vi "DHE_Get.vi"(0 "refnum":i32, 1 "DHE_DBSRef":T1, 2 "Command + switches":string, 5 "Command":string, 7 "physical unit":string, 9 "swhitches":string[](array[string]), 11 "error in (no error)":errorcluster) -> (4 "refnum out":i32, 6 "response":string, 15 "error out":errorcluster)   [LabVIEW 2016]
uses:
  Common/public/vis/CMN_TimingInfo.ctl
  DBSHAND/private/vis/DatabaseHand_RefNum.ctl
  DBSHAND/private/vis/DatabaseHand_Element_Get(string).vi
  DBSHAND/private/vis/DatabaseHand_Element_Get(U32).vi
  DBSHAND/private/vis/DatabaseHand_Element_Get(bool).vi
  DBSHAND/private/vis/DatabaseHand_Element_Get(double).vi
  DBSHAND/private/vis/DatabaseHand_Element_Set(I32).vi
  DBSHAND/private/vis/DatabaseHand_Element_Get(I32).vi
panel:
  out "Timing":T2={"PixelTime"=1.0, "SkipPixel"=1.0, "SkipRow"=1.0, "ShiftRow"=1.0, "ShiftedPix"=1, "known_overhead"=1.0, "DET_READ_TIME"=1.0} {"DET_READ_TIME" format="%.2f"; "known_overhead" format="%.2f"; "ShiftRow" format="%.2f"; "SkipRow" format="%.2f"; "SkipPixel" format="%.2f"; "PixelTime" format="%.2f"}
  out "ControllerConfigCluster":T3
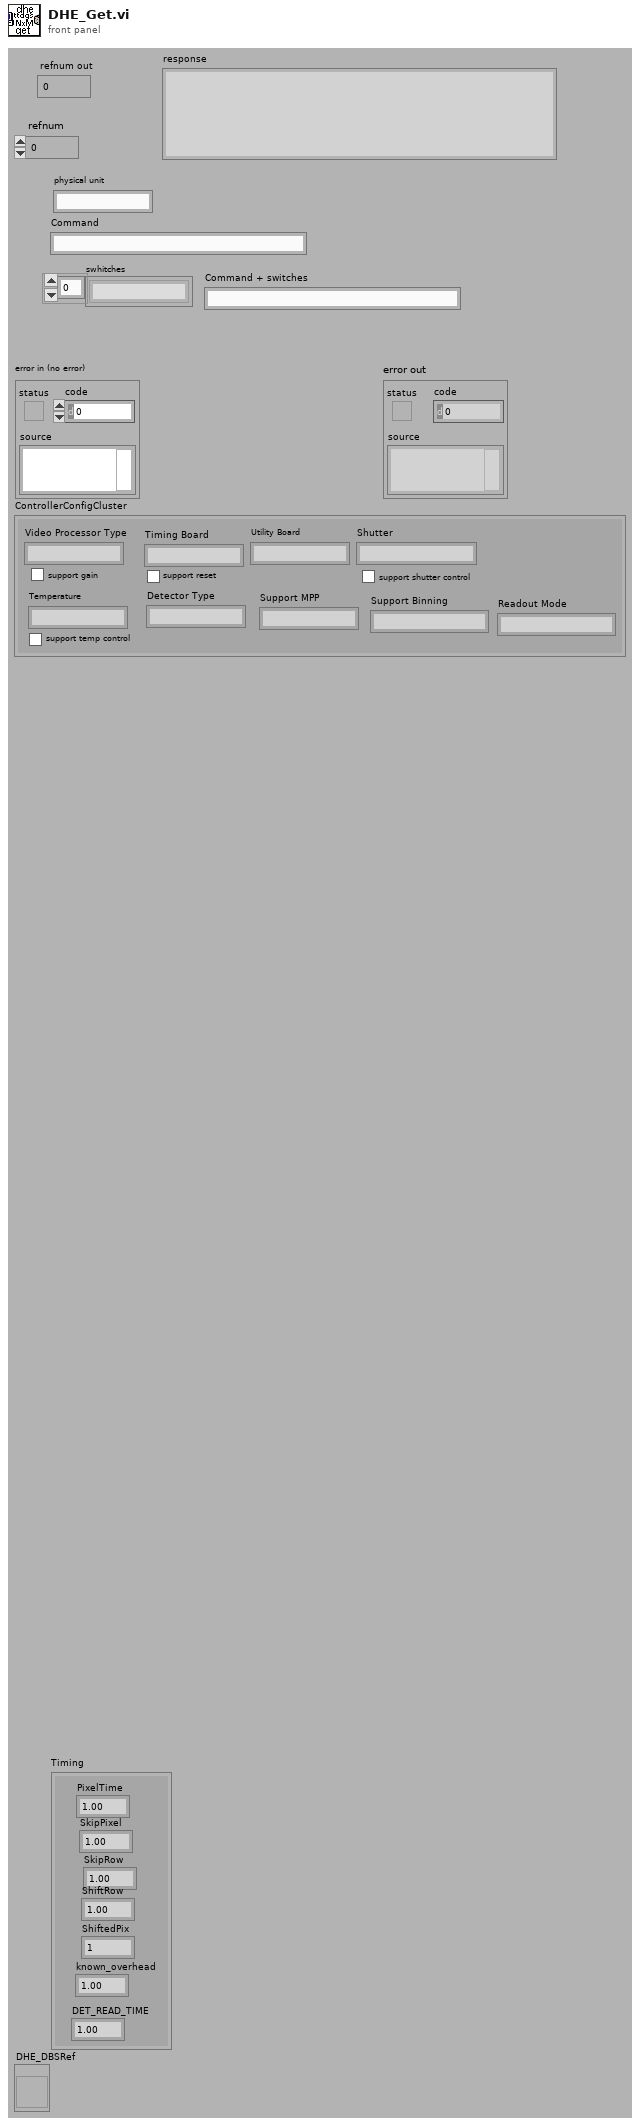
[diagram p1: front panel]
types:
  T1 = typedef "DatabaseHand_RefNum.ctl" = refnum<vi>
  T2 = typedef "CMN_TimingInfo.ctl" = cluster{"PixelTime":sgl, "SkipPixel":sgl, "SkipRow":sgl, "ShiftRow":sgl, "ShiftedPix":u16, "known_overhead":sgl, "DET_READ_TIME":sgl}
  T3 = cluster{"Video Processor Type":string, "support gain":bool, "Timing Board":string, "support reset":bool, "Utility Board":string, "Shutter":string, "Temperature":string, "support temp control":bool, "Detector Type":string, "Support MPP":string, "Support Binning":string, "Readout Mode":string, "support shutter control":bool}
  T4 = enum16{"add", "delete", "find", "clear all", "getall"}
  T5 = typedef "CMN_ContStatus.ctl" = cluster{"Response":string, "power":bool, "shutter":bool, "artifdata":bool, "idlemode":bool, "reset":bool, "gain":u8, "speed":u8, "resetPCI":bool, "autoshutter":bool, "TempSetPoint":i32, "multipleextensions":bool, "displayImage":bool, "coadding":bool, "images being coadded":i32, "Operation Mode":enum16{"normal", "coadd", "fawler"}, "frames to write":cluster{"subs":bool, "reset":bool, "exposed":bool}, "fawler samples":i32, "write auto":bool, "datatype":string, "frames to display":cluster{"subs":bool, "reset":bool, "exposed":bool}, "sur":i32, "autoclear":bool}
  T6 = typedef "DHE_Obs.ctl" = cluster{"observer":string, "obstype":string, "exptime":dbl, "coadds":i32, "fowler":i32, "nimages":i32, "display":bool, "autowrite":bool, "frames to write":cluster{"subs":bool, "reset":bool, "exposed":bool}, "frames to display":cluster{"subs":bool, "reset":bool, "exposed":bool}, "sur":i32}
  T7 = typedef "DHE_Img.ctl" = cluster{"title":string, "comment":string, "rootname":string, "imnumber":i32, "mext":bool, "imdir":string, "basename":string, "imprefix":string, "imsufix":string, "froot":string}
  T8 = typedef "GEOM_AmpModifiers.ctl" = cluster{"Binning":T9, "sections":T10[]}
  T9 = typedef "GEOM_Binning.ctl" = cluster{"x":u32, "y":u32}
  T10 = typedef "GEOM_Moifier.ctl" = cluster{"name":string, "header section":string, "comment":string, "value":i32, "binning?":bool, "Where":enum16{"predata", "postdata"}, "add In":enum16{"columns", "rows", "none"}}
  T11 = enum16{"Idle", "Exposing", "Paused", "AbortExp", "Reading", "AbortRead", "FinishedReading", "Resetting", "Reducing", "Initializing"}
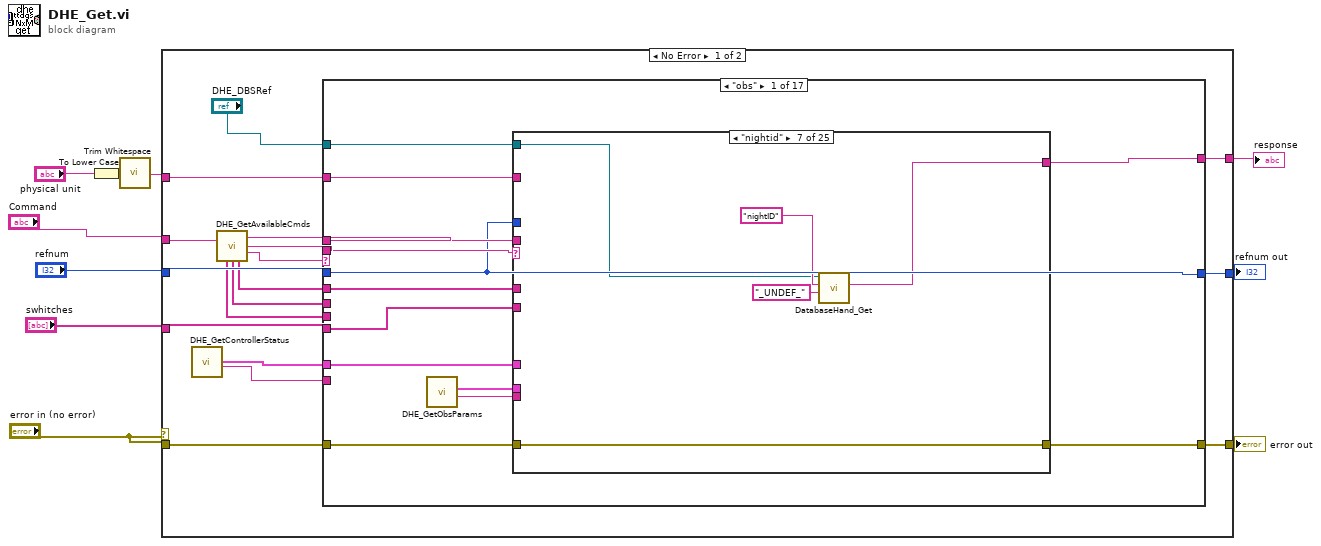
[diagram p0: block diagram]
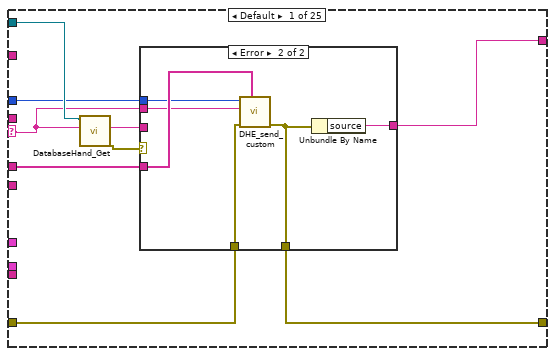
[diagram p2: hidden frame]
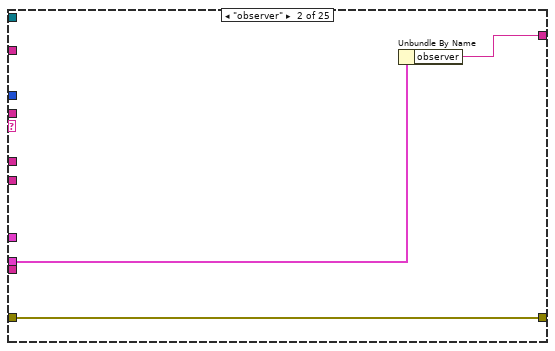
[diagram p4: hidden frame]
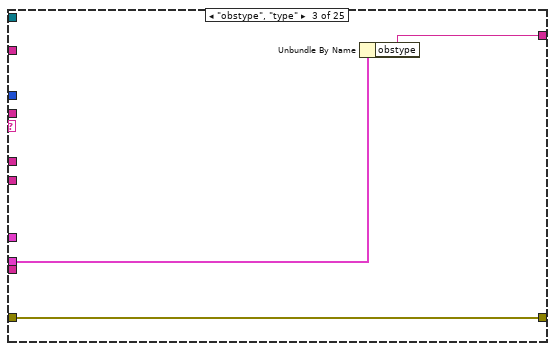
[diagram p5: hidden frame]
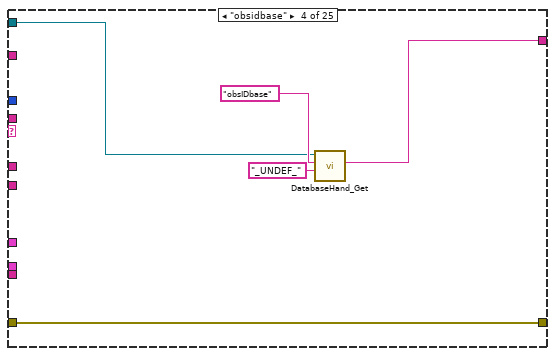
[diagram p6: hidden frame]
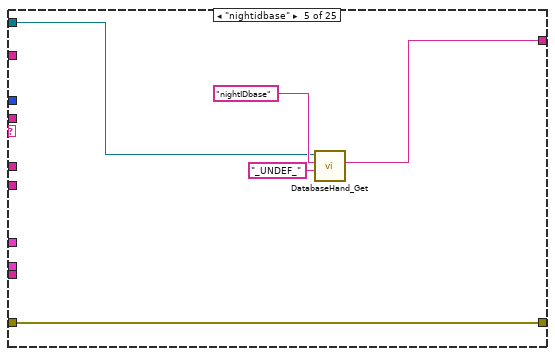
[diagram p7: hidden frame]
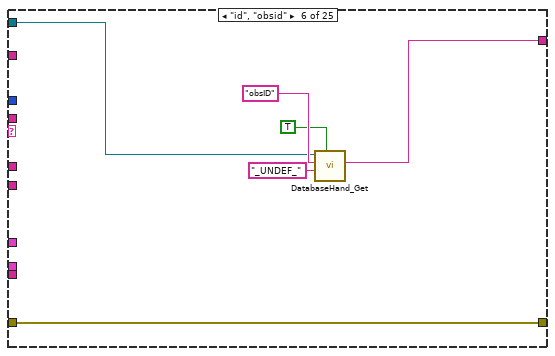
[diagram p8: hidden frame]
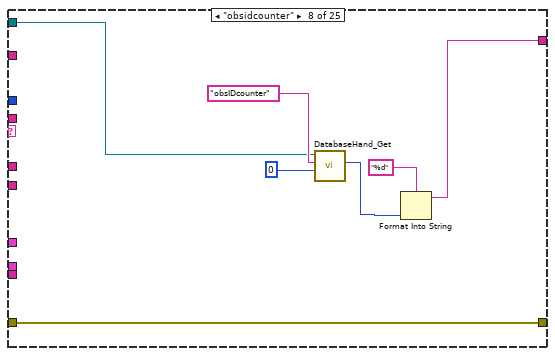
[diagram p9: hidden frame]
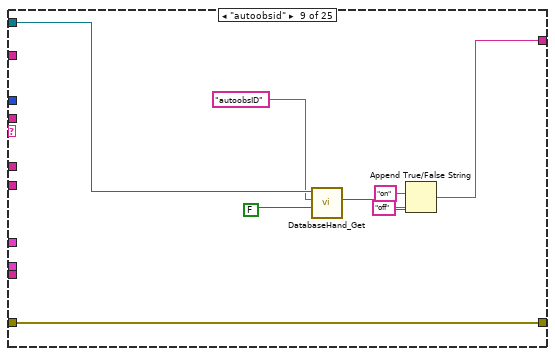
[diagram p10: hidden frame]
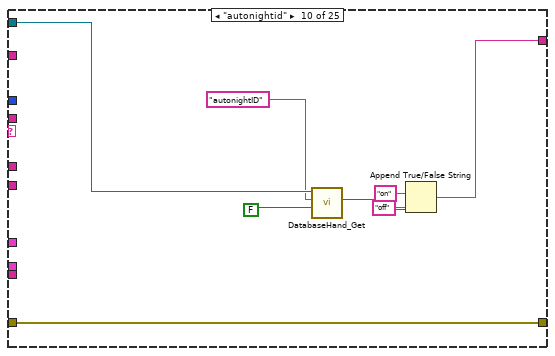
[diagram p11: hidden frame]
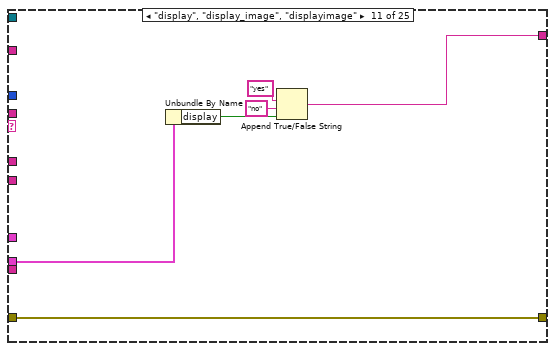
[diagram p12: hidden frame]
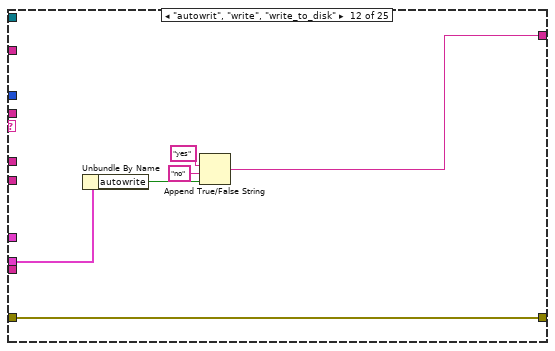
[diagram p13: hidden frame]
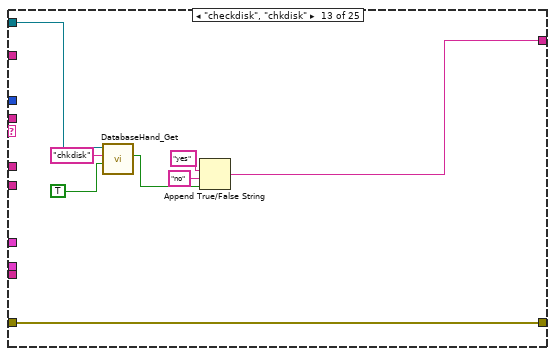
[diagram p14: hidden frame]
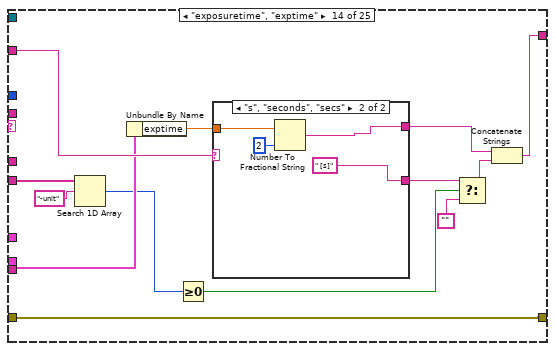
[diagram p15: hidden frame]
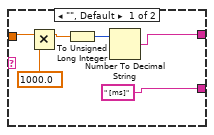
[diagram p16: hidden frame]
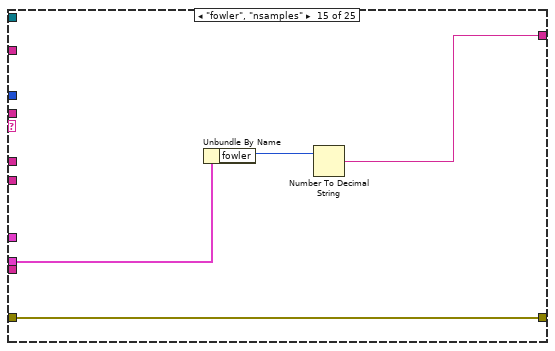
[diagram p17: hidden frame]
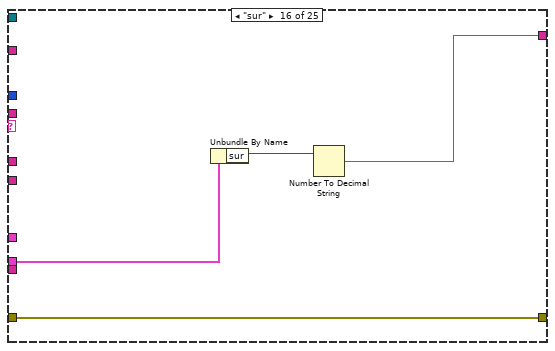
[diagram p18: hidden frame]
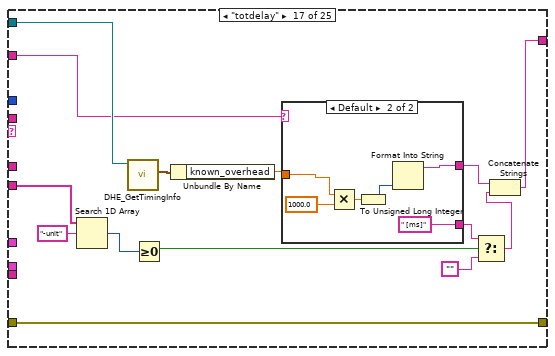
[diagram p19: hidden frame]
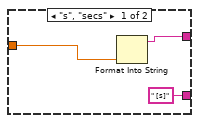
[diagram p20: hidden frame]
diagram:
  n1 = To Lower Case(string="physical unit") -> (all lower case string=w5:string)
  n2 = call <vilib>:"Trim Whitespace.vi"("string"=w5) -> ("trimmed string"=w1:string)  [unwired: 1 in]
  n3 = case shown="No Error" "error in (no error)" {
    tunnel: "error in (no error)" -> [w27 w945]
    tunnel: [w26 w945] -> w8
    tunnel: "refnum" -> [w25 w946]
    tunnel: [w24 w946] -> w10
    tunnel: "Command" -> [w19 _]
    tunnel: w1 -> [w22 _]
    tunnel: [w21 w944] -> w4
    tunnel: "swhitches" -> [w20 _]
    frame No Error {
      n4 = call "DHE_GetControllerStatus.vi"() -> ("dhe string"=w12:string, "ControllerStatus"=w23:T5)  [unwired: 10 out]
      n5 = call "DHE_GetAvailableCmds.vi"("input command"=w19) -> ("remaining"=w18:string, "field"=w16:string, "parent"=w17:string, "SDSU_image_cmds out"=w15:string[], "SDSU_dhe_cmds out"=w14:string[], "SDSU_obs_cmds out"=w13:string[])  [unwired: 9 out]
      n6 = case shown="\"obs\"" w17 {
        selector: w17 -> [_ _ _ _ _ _ _ _ _ _ _ _ _ _ _ _ w911]
        tunnel: w27 -> [w36 w261 w418 w759 w797 w802 w808 w812 w823 w841 w845 w851 w855 w864 w871 w875 w924]
        tunnel: [w35 w260 w417 w759 w797 w802 w808 w812 w822 w838 w844 w851 w855 w864 w871 w874 w923] -> w26
        tunnel: w25 -> [w29 w253 w408 w758 w796 w805 w809 w813 w821 w840 w846 w853 w854 w863 w870 w881 w921]
        tunnel: [w29 w253 w408 w758 w796 w805 w809 w813 w821 w840 w846 w853 w854 w863 w870 w881 w920] -> w24
        tunnel: w18 -> [w33 w262 w411 _ _ _ _ _ _ w837 _ w848 _ _ _ w884 w918]
        tunnel: w23 -> [w38 w259 w413 _ _ _ _ _ _ _ _ _ _ _ _ _ _]
        tunnel: w22 -> [w34 w258 _ _ _ _ _ _ _ _ _ _ _ _ _ _ _]
        tunnel: [w39 w265 w416 w757 w798 w801 w807 w811 w814 w839 w842 w852 w856 w859 w868 w876 w922] -> w21
        tunnel: w20 -> [w28 w254 w412 _ _ _ _ _ w820 _ _ _ _ _ _ w880 _]
        tunnel: w16 -> [w40 w264 w415 _ _ _ _ _ _ _ _ _ _ _ _ _ _]
        tunnel: w15 -> [_ w263 _ _ _ _ _ _ _ _ _ _ _ _ _ _ _]
        tunnel: w14 -> [_ _ w414 _ _ _ _ _ _ _ _ _ _ _ _ _ _]
        tunnel: w13 -> [w37 _ _ _ _ _ _ _ _ _ _ _ _ _ _ _ _]
        tunnel: w12 -> [_ _ w410 _ _ _ _ _ _ _ _ _ _ _ _ _ _]
        tunnel: "DHE_DBSRef" -> [w30 w255 w409 _ _ _ _ _ _ _ _ _ _ w867 w873 _ w919]
        frame "obs" {
          n7 = call "DHE_GetObsParams.vi"() -> ("obs string"=w31:string, "DHE_OBS"=w32:T6)  [unwired: 10 out]
          n8 = case shown="\"nightid\"" w40 {
            selector: w40 -> [w42 _ _ _ _ _ _ _ _ _ _ _ _ _ _ _ _ _ _ _ _ _ _ _ _]
            tunnel: [w48 w58 w61 w64 w69 w75 w80 w85 w94 w102 w110 w116 w125 w130 w153 w157 w163 w186 w208 w228 w233 w236 w237 w244 w251] -> w39
            tunnel: w38 -> [_ _ _ _ _ _ _ _ _ _ _ _ _ _ _ _ _ _ _ _ _ _ w242 w249 _]
            tunnel: w37 -> [w49 _ _ _ _ _ _ _ _ _ _ _ _ _ _ _ _ _ _ _ _ _ _ _ _]
            tunnel: w36 -> [w47 w60 w63 w65 w70 w76 w81 w89 w93 w101 w109 w115 w124 w139 w152 w156 w171 w194 w216 w227 w232 w235 w243 w250 w252]
            tunnel: [w46 w60 w63 w65 w70 w76 w81 w89 w93 w101 w109 w115 w124 w139 w152 w156 w171 w194 w216 w227 w232 w234 w243 w250 w252] -> w35
            tunnel: w34 -> [_ _ _ _ _ _ _ _ _ _ _ _ _ w140 _ _ w168 w191 w213 _ _ _ _ _ _]
            tunnel: w33 -> [_ _ _ _ _ _ _ _ _ _ _ _ _ _ _ _ _ _ _ _ _ _ _ _ _]
            tunnel: w32 -> [_ w59 w62 _ _ _ _ _ _ _ w108 w114 _ w138 w151 w155 _ _ _ w226 w231 _ _ _ _]
            tunnel: w31 -> [_ _ _ _ _ _ _ _ _ _ _ _ _ _ _ _ _ _ _ _ _ _ _ _ w251]
            tunnel: w30 -> [w44 _ _ w66 w71 w77 w82 w90 w95 w103 _ _ w123 _ _ _ w172 _ _ _ _ _ _ _ _]
            tunnel: w29 -> [w41 _ _ _ _ _ _ _ _ _ _ _ _ _ _ _ _ w193 w215 _ _ _ _ _ _]
            tunnel: w28 -> [_ _ _ _ _ _ _ _ _ _ _ _ _ w136 _ _ w166 w188 w210 _ _ _ _ _ _]
            frame Default {
              n9 = call-poly "DatabaseHand_Get.vi"("name"=w42, "Database RefNum in"=w44) -> ("error out"=w45:errorcluster, "value"=w43:string)  [unwired: 3 in, 5 out]
              n10 = case shown="Error" w45 {
                tunnel: w49 -> [_ w57]
                tunnel: [w50 w56] -> w48
                tunnel: w47 -> [w51 w55]
                tunnel: [w51 w54] -> w46
                tunnel: w42 -> [_ w53]
                tunnel: w43 -> [w50 _]
                tunnel: w41 -> [_ w52]
                frame No Error {
                }
                frame Error {
                  n11 = call "DHE_send_custom.vi"("valid params"=w57, "error in (no error)"=w55, "args"=w53, "fd"=w52) -> ("error IO"=w54:errorcluster)  [unwired: 7 out]
                  n12 = Unbundle By Name(w54) -> ("source"=w56:string)
                }
              }
            }
            frame "observer" {
              n13 = Unbundle By Name(w59) -> ("observer"=w58:string)
            }
            frame "obstype", "type" {
              n14 = Unbundle By Name(w62) -> ("obstype"=w61:string)
            }
            frame "obsidbase" {
              n15 = call-poly "DatabaseHand_Get.vi"("default value"="_UNDEF_", "name"="obsIDbase" ("value"), "Database RefNum in"=w66) -> ("value"=w64:string)  [unwired: 2 in, 6 out]
            }
            frame "nightidbase" {
              n16 = call-poly "DatabaseHand_Get.vi"("default value"="_UNDEF_", "name"="nightIDbase" ("value"), "Database RefNum in"=w71) -> ("value"=w69:string)  [unwired: 2 in, 6 out]
            }
            frame "id", "obsid" {
              n17 = call-poly "DatabaseHand_Get.vi"("nd queue"=TRUE, "default value"="_UNDEF_", "name"="obsID" ("value"), "Database RefNum in"=w77) -> ("value"=w75:string)  [unwired: 1 in, 6 out]
            }
            frame "nightid" {
              n18 = call-poly "DatabaseHand_Get.vi"("default value"="_UNDEF_", "name"="nightID" ("value"), "Database RefNum in"=w82) -> ("value"=w80:string)  [unwired: 2 in, 6 out]
            }
            frame "obsidcounter" {
              n19 = call-poly "DatabaseHand_Get.vi"("default value"=u32 0, "name"="obsIDcounter" ("value"), "Database RefNum in"=w90) -> ("value"=w86:u32)  [unwired: 2 in, 6 out]
              n20 = Format Into String(format string="%d", w86) -> (resulting string=w85:string)  [unwired: 2 in, 1 out]
            }
            frame "autoobsid" {
              n21 = call-poly "DatabaseHand_Get.vi"("default value"=FALSE, "name"="autoobsID", "Database RefNum in"=w95) -> ("value"=w98:bool)  [unwired: 2 in, 6 out]
              n22 = Append True/False String(1:w98, 2:"off" ("false string"), 3:"on" ("true string")) -> (0:w94:string)  [unwired: 1 out]
            }
            frame "autonightid" {
              n23 = call-poly "DatabaseHand_Get.vi"("default value"=FALSE, "name"="autonightID", "Database RefNum in"=w103) -> ("value"=w106:bool)  [unwired: 2 in, 6 out]
              n24 = Append True/False String(1:w106, 2:"off" ("false string"), 3:"on" ("true string")) -> (0:w102:string)  [unwired: 1 out]
            }
            frame "display", "display_image", "displayimage" {
              n25 = Unbundle By Name(w108) -> ("display"=w113:bool)
              n26 = Append True/False String(1:w113, 2:"no" ("false string"), 3:"yes" ("true string")) -> (0:w110:string)  [unwired: 1 out]
            }
            frame "autowrit", "write", "write_to_disk" {
              n27 = Unbundle By Name(w114) -> ("autowrite"=w119:bool)
              n28 = Append True/False String(1:w119, 2:"no" ("false string"), 3:"yes" ("true string")) -> (0:w116:string)  [unwired: 1 out]
            }
            frame "checkdisk", "chkdisk" {
              n29 = call-poly "DatabaseHand_Get.vi"("default value"=TRUE, "name"="chkdisk", "Database RefNum in"=w123) -> ("value"=w120:bool)  [unwired: 2 in, 6 out]
              n30 = Append True/False String(1:w120, 2:"no" ("false string"), 3:"yes" ("true string")) -> (0:w125:string)  [unwired: 1 out]
            }
            frame "exposuretime", "exptime" {
              n31 = Search 1D Array(1D array=w136, element="-unit") -> (index of element=w134:i32)  [unwired: 1 out]
              n32 = Unbundle By Name(w138) -> ("exptime"=w137:dbl)
              n33 = Greater Or Equal To 0?(x=w134) -> (x >= 0?=w133:bool)
              n34 = case shown="\"s\", \"seconds\", \"secs\"" w140 {
                tunnel: [w142 w148] -> w129
                tunnel: w137 -> [w146 w150]
                tunnel: [" [ms]" ("string") " [s]" ("string")] -> w128
                frame "", Default {
                  n35 = Multiply(x=w146, y=1000.0) -> (x*y=w143:dbl)
                  n36 = To Unsigned Long Integer(number=w143) -> (unsigned 32bit integer=w144:u32)
                  n37 = Number To Decimal String(number=w144) -> (decimal integer string=w142:string)  [unwired: 1 out]
                }
                frame "s", "seconds", "secs" {
                  n38 = Number To Fractional String(number=w150, precision (6)=i16 2) -> (F-format string=w148:string)  [unwired: 2 out]
                }
              }
              n39 = Select(t=w128, s=w133, f="") -> (s? t:f=w131:string)
              n40 = Concatenate Strings(w129, w131) -> (w130:string)
            }
            frame "fowler", "nsamples" {
              n41 = Unbundle By Name(w151) -> ("fowler"=w154:i32)
              n42 = Number To Decimal String(number=w154) -> (decimal integer string=w153:string)  [unwired: 1 out]
            }
            frame "sur" {
              n43 = Unbundle By Name(w155) -> ("sur"=w158:i32)
              n44 = Number To Decimal String(number=w158) -> (decimal integer string=w157:string)  [unwired: 1 out]
            }
            frame "totdelay" {
              n45 = Search 1D Array(1D array=w166, element="-unit") -> (index of element=w165:i32)  [unwired: 1 out]
              n46 = call "DHE_GetTimingInfo.vi"("Database RefNum out"=w172) -> ("Timing"=w170:T2)  [unwired: 10 out]
              n47 = Greater Or Equal To 0?(x=w165) -> (x >= 0?=w162:bool)
              n48 = Unbundle By Name(w170) -> ("known_overhead"=w169:sgl)
              n49 = case shown="Default" w168 {
                tunnel: [w175 w181] -> w164
                tunnel: w169 -> [w174 w180]
                tunnel: [" [s]" " [ms]"] -> w160
                frame "s", "secs" {
                  n50 = Format Into String(w174) -> (resulting string=w175:string)  [unwired: 3 in, 1 out]
                }
                frame Default {
                  n51 = Multiply(x=w180, y=sgl 1000.0) -> (x*y=w179:sgl)
                  n52 = To Unsigned Long Integer(number=w179) -> (unsigned 32bit integer=w178:u32)
                  n53 = Format Into String(w178) -> (resulting string=w181:string)  [unwired: 3 in, 1 out]
                }
              }
              n54 = Select(t=w160, s=w162, f="") -> (s? t:f=w159:string)
              n55 = Concatenate Strings(w164, w159) -> (w163:string)
            }
            frame "intdelay" {
              n56 = Search 1D Array(1D array=w188, element="-unit") -> (index of element=w189:i32)  [unwired: 1 out]
              n57 = Greater Or Equal To 0?(x=w189) -> (x >= 0?=w185:bool)
              n58 = call "DHE_get_intdelay.vi"("fd in"=w193) -> ("msdelay"=w192:sgl)  [unwired: 1 in, 13 out]
              n59 = case shown="Default" w191 {
                tunnel: [w196 w203] -> w187
                tunnel: w192 -> [w199 w202]
                tunnel: [" [s]" ("t") " [ms]" ("t")] -> w182
                frame "s", "secs" {
                  n60 = Divide(x=w199, y=sgl 1000.0) -> (x/y=w197:sgl)
                  n61 = Format Into String(w197) -> (resulting string=w196:string)  [unwired: 3 in, 1 out]
                }
                frame Default {
                  n62 = To Unsigned Long Integer(number=w202) -> (unsigned 32bit integer=w201:u32)
                  n63 = Format Into String(w201) -> (resulting string=w203:string)  [unwired: 3 in, 1 out]
                }
              }
              n64 = Select(t=w182, s=w185, f="") -> (s? t:f=w183:string)
              n65 = Concatenate Strings(w187, w183) -> (w186:string)
            }
            frame "seqdelay" {
              n66 = Search 1D Array(1D array=w210, element="-unit") -> (index of element=w211:i32)  [unwired: 1 out]
              n67 = Greater Or Equal To 0?(x=w211) -> (x >= 0?=w205:bool)
              n68 = call "DHE_get_seqdelay.vi"("fd in"=w215) -> ("idle"=w214:sgl)  [unwired: 1 in, 13 out]
              n69 = case shown="Default" w213 {
                tunnel: [w218 w225] -> w209
                tunnel: w214 -> [w221 w224]
                tunnel: [" [s]" " [ms]"] -> w207
                frame "s", "secs" {
                  n70 = Divide(x=w221, y=sgl 1000.0) -> (x/y=w219:sgl)
                  n71 = Format Into String(w219) -> (resulting string=w218:string)  [unwired: 3 in, 1 out]
                }
                frame Default {
                  n72 = To Unsigned Long Integer(number=w224) -> (unsigned 32bit integer=w223:u32)
                  n73 = Format Into String(w223) -> (resulting string=w225:string)  [unwired: 3 in, 1 out]
                }
              }
              n74 = Select(t=w207, s=w205, f="") -> (s? t:f=w204:string)
              n75 = Concatenate Strings(w209, w204) -> (w208:string)
            }
            frame "coadds" {
              n76 = Unbundle By Name(w226) -> ("coadds"=w229:i32)
              n77 = Number To Decimal String(number=w229) -> (decimal integer string=w228:string)  [unwired: 1 out]
            }
            frame "imagestoread", "nimages", "numreads" {
              n78 = Unbundle By Name(w231) -> ("nimages"=w230:i32)
              n79 = Number To Decimal String(number=w230) -> (decimal integer string=w233:string)  [unwired: 1 out]
            }
            frame "roi" {
              n80 = call "GEOM_GetROI.vi"("error in (no error)"=w235) -> ("error out"=w234:errorcluster, "Requested ROI"=w236:string)  [unwired: 9 out]
            }
            frame "writeframes" {
              n81 = Unbundle By Name(w242) -> ("frames to write.subs"=w240:bool, "frames to write.reset"=w239:bool, "frames to write.exposed"=w238:bool)
              n82 = Format Into String(format string="subs=%s, reset=%s, expo=%s", w240, w239, w238) -> (resulting string=w237:string)  [unwired: 2 in, 1 out]
            }
            frame "dispframes" {
              n83 = Unbundle By Name(w249) -> ("frames to display.subs"=w247:bool, "frames to display.reset"=w246:bool, "frames to display.exposed"=w245:bool)
              n84 = Format Into String(format string="subs=%s, reset=%s, expo=%s", w247, w246, w245) -> (resulting string=w244:string)  [unwired: 2 in, 1 out]
            }
            frame "" {
            }
          }
        }
        frame "image" {
          n85 = call "DHE_GetImageParams.vi"() -> ("image string"=w256:string, "DHE_IMAGE"=w257:T7)  [unwired: 10 out]
          n86 = case shown="\"expid\"" w264 {
            selector: w264 -> [w270 _ _ _ _ _ _ _ _ _ _ _ _ _ _ _ _ _ _ _ _]
            tunnel: [w271 w283 w288 w294 w297 w315 w320 w327 w330 w333 w340 w350 w353 w356 w362 w366 w374 w380 w385 w391 w406] -> w265
            tunnel: w263 -> [w274 _ _ _ _ _ _ _ _ _ _ _ _ _ _ _ _ _ _ _ _]
            tunnel: w262 -> [_ _ _ _ _ _ _ _ _ _ _ _ _ _ _ _ _ _ _ w389 _]
            tunnel: w261 -> [w273 w285 w287 w293 w303 w318 w324 w329 w332 w335 w342 w352 w355 w358 w361 w365 w373 w378 w387 w393 w407]
            tunnel: [w272 w285 w287 w293 w303 w318 w324 w329 w332 w335 w342 w352 w355 w358 w361 w365 w373 w378 w386 w392 w407] -> w260
            tunnel: w259 -> [_ _ _ _ _ _ _ _ _ _ _ _ _ _ _ _ _ _ _ _ _]
            tunnel: w258 -> [_ _ _ _ w301 _ _ _ _ _ _ _ _ _ _ _ _ w379 _ _ _]
            tunnel: w257 -> [_ w284 _ _ _ _ _ w328 w331 w334 w341 w351 w354 w357 w360 w364 _ _ _ _ _]
            tunnel: w256 -> [_ _ _ _ _ _ _ _ _ _ _ _ _ _ _ _ _ _ _ _ w406]
            tunnel: w255 -> [w267 _ w290 w296 w304 w319 w326 _ _ _ _ _ _ _ _ _ w371 w377 _ _ _]
            tunnel: w254 -> [_ _ _ _ _ _ _ _ _ _ w339 _ _ _ _ _ _ _ w381 _ _]
            tunnel: w253 -> [w266 _ _ _ _ _ _ _ _ _ _ _ _ _ _ _ _ _ _ _ _]
            frame Default {
              n87 = call-poly "DatabaseHand_Get.vi"("name"=w270, "Database RefNum in"=w267) -> ("error out"=w269:errorcluster, "value"=w268:string)  [unwired: 3 in, 5 out]
              n88 = case shown="Error" w269 {
                tunnel: w274 -> [_ w282]
                tunnel: w273 -> [w275 w281]
                tunnel: [w275 w280] -> w272
                tunnel: [w276 w279] -> w271
                tunnel: w270 -> [_ w278]
                tunnel: w268 -> [w276 _]
                tunnel: w266 -> [_ w277]
                frame No Error {
                }
                frame Error {
                  n89 = call "DHE_send_custom.vi"("valid params"=w282, "error in (no error)"=w281, "args"=w278, "fd"=w277) -> ("error IO"=w280:errorcluster)  [unwired: 7 out]
                  n90 = Unbundle By Name(w280) -> ("source"=w279:string)
                }
              }
            }
            frame "imagetitle", "title" {
              n91 = Unbundle By Name(w284) -> ("title"=w283:string)
            }
            frame "expidbase" {
              n92 = call-poly "DatabaseHand_Get.vi"("default value"="_UNDEF_", "name"="expIDbase" ("value"), "Database RefNum in"=w290) -> ("value"=w288:string)  [unwired: 2 in, 6 out]
            }
            frame "expid" {
              n93 = call-poly "DatabaseHand_Get.vi"("nd queue"=TRUE, "default value"="_UNDEF_", "name"="expID" ("value"), "Database RefNum in"=w296) -> ("value"=w294:string)  [unwired: 1 in, 6 out]
            }
            frame "integrationtime", "integtime" {
              n94 = call "DHE_GetObsParams.vi"() -> ("DHE_OBS"=w302:T6)  [unwired: 11 out]
              n95 = Unbundle By Name(w302) -> ("exptime"=w300:dbl)
              n96 = call-poly "DatabaseHand_Get.vi"("default value"=w300, "name"="rintegtime", "Database RefNum in"=w304) -> ("value"=w299:dbl)  [unwired: 2 in, 6 out]
              n97 = case shown="\"s\", \"sec\", \"secs\"" w301 {
                tunnel: w299 -> [w309 w311]
                tunnel: [w305 w310] -> w297
                frame Default {
                  n98 = Multiply(x=1000.0, y=w309) -> (x*y=w307:dbl)
                  n99 = Format Into String(format string="%d", w307) -> (resulting string=w305:string)  [unwired: 2 in, 1 out]
                }
                frame "s", "sec", "secs" {
                  n100 = Format Into String(w311) -> (resulting string=w310:string)  [unwired: 3 in, 1 out]
                }
              }
            }
            frame "autoexpid" {
              n101 = call-poly "DatabaseHand_Get.vi"("default value"=TRUE, "name"="autoexpID", "Database RefNum in"=w319) -> ("value"=w316:bool)  [unwired: 2 in, 6 out]
              n102 = Append True/False String(1:w316, 2:"off" ("false string"), 3:"on" ("true string")) -> (0:w315:string)  [unwired: 1 out]
            }
            frame "expidcounter" {
              n103 = call-poly "DatabaseHand_Get.vi"("default value"=u32 0, "name"="expIDcounter" ("value"), "Database RefNum in"=w326) -> ("value"=w321:u32)  [unwired: 2 in, 6 out]
              n104 = Format Into String(format string="%d", w321) -> (resulting string=w320:string)  [unwired: 2 in, 1 out]
            }
            frame "comment", "imagecomment" {
              n105 = Unbundle By Name(w328) -> ("comment"=w327:string)
            }
            frame "rootname" {
              n106 = Unbundle By Name(w331) -> ("rootname"=w330:string)
            }
            frame "basename" {
              n107 = Unbundle By Name(w334) -> ("basename"=w333:string)
            }
            frame "dir", "directory" {
              n108 = Search 1D Array(1D array=w339, element="-full") -> (index of element=w337:i32)  [unwired: 1 out]
              n109 = Greater Or Equal To 0?(x=w337) -> (x >= 0?=w336:bool)
              n110 = case shown="True" w336 {
                tunnel: w341 -> [w344 w349]
                tunnel: [w343 w346] -> w340
                frame False {
                  n111 = Unbundle By Name(w344) -> ("imdir"=w343:string)
                }
                frame True {
                  n112 = Unbundle By Name(w349) -> ("imdir"=w348:string, "froot"=w347:string)
                  n113 = call "DHE_BuildRootname.vi"("froot"=w347, "imdir"=w348) -> ("rootpath"=w345:path)  [unwired: 4 in, 4 out]
                  n114 = Path To String(path=w345) -> (string=w346:string)
                }
              }
            }
            frame "fixed_root", "froot" {
              n115 = Unbundle By Name(w351) -> ("froot"=w350:string)
            }
            frame "imprefix", "prefix" {
              n116 = Unbundle By Name(w354) -> ("imprefix"=w353:string)
            }
            frame "imsufix", "sufix" {
              n117 = Unbundle By Name(w357) -> ("imsufix"=w356:string)
            }
            frame "imagenumber", "imnumber", "number" {
              n118 = Unbundle By Name(w360) -> ("imnumber"=w359:i32)
              n119 = Number To Decimal String(number=w359) -> (decimal integer string=w362:string)  [unwired: 1 out]
            }
            frame "extensions", "mext", "multipleextensions" {
              n120 = Unbundle By Name(w364) -> ("mext"=w363:bool)
              n121 = Append True/False String(1:w363, 2:"no" ("false string"), 3:"yes" ("true string")) -> (0:w366:string)  [unwired: 1 out]
            }
            frame "detext" {
              n122 = call-poly "DatabaseHand_Get.vi"("default value"=FALSE, "name"="detext" ("value"), "Database RefNum in"=w371) -> ("value"=w369:bool)  [unwired: 2 in, 6 out]
              n123 = Append True/False String(1:w369, 2:"no" ("false string"), 3:"yes" ("true string")) -> (0:w374:string)  [unwired: 1 out]
            }
            frame "progress" {
              n124 = call "DHE_GetProgress.vi"("phys. unit"=w379, "Databse Ref"=w377) -> ("progress"=w380:string)  [unwired: 9 out]
            }
            frame "geometry" {
              n125 = Search 1D Array(1D array=w381, element="-full") -> (index of element=w383:i32)  [unwired: 1 out]
              n126 = Less Than 0?(x=w383) -> (x < 0?=w382:bool)
              n127 = call "DHE_GetGeometry.vi"("error in (no error)"=w387, "binned?"=w382) -> ("error out"=w386:errorcluster, "geometry"=w385:string)  [unwired: 8 out]
            }
            frame "modifiers" {
              n128 = Scan From String(format string="%s", input string=w389) -> (output 1=w390:string)  [unwired: 2 in, 4 out]
              n129 = case shown="\"order\", \"xorder\", \"yorder\"" w390 {
                selector: w390 -> [w399 _]
                tunnel: w393 -> [w397 w405]
                tunnel: [w396 w404] -> w392
                tunnel: [w394 w403] -> w391
                frame "order", "xorder", "yorder" {
                  n130 = Concatenate Strings("GET " ("string"), w399) -> (w398:string)
                  n131 = call "CMN_toUnsc.vi"("responseQ"="dhe2unsc", "ms timeout (-1)"=5000, "error in (no error)"=w397, "command"=w398) -> ("error out"=w396:errorcluster, "response"=w395:errorcluster)  [unwired: 5 in, 1 out]
                  n132 = Unbundle By Name(w395) -> ("source"=w394:string)
                }
                frame Default {
                  n133 = call "DHE_GetModifiersInfo.vi"("error in (no error)"=w405) -> ("error out"=w404:errorcluster, "modifiers"=w403:string)  [unwired: 9 out]
                }
              }
            }
            frame "" {
            }
          }
        }
        frame "dhe" {
          n134 = case shown="\"min_exptime\", \"minexptime\"" w415 {
            selector: w415 -> [w420 _ _ _ _ _ _ _ _ _ _ _ _ _ _ _ _ _ _ _ _ _ _ _ _ _ _ _ _ _ _ _ _ _]
            tunnel: w418 -> [w427 w441 w444 w446 w448 w449 w455 w467 w496 w498 w514 w517 w527 w540 w545 w552 w557 w561 w566 w569 w583 w588 w603 w611 w616 w622 w626 w630 w644 w688 w706 w728 w735 w748]
            tunnel: [w426 w440 w444 w446 w448 w449 w455 w467 w496 w498 w514 w517 w527 w540 w545 w552 w557 w561 w566 w569 w582 w588 w603 w611 w616 w621 w625 w630 w644 w688 w706 w727 w735 w748] -> w417
            tunnel: [w425 w435 w442 w445 w447 w452 w456 w468 w493 w497 w503 w516 w526 w539 w544 w551 w556 w560 w563 w573 w581 w591 w604 w612 w615 w623 w627 w629 w636 w670 w709 w717 w738 w747] -> w416
            tunnel: w414 -> [w424 _ _ _ _ _ _ _ _ _ _ _ _ _ _ _ _ _ _ _ _ _ _ _ _ _ _ _ _ _ _ _ _ _]
            tunnel: w413 -> [_ _ _ _ _ w451 w457 w469 _ w499 _ w518 _ w541 w546 _ _ _ _ w572 _ w590 _ _ _ _ _ _ _ _ _ _ _ _]
            tunnel: w412 -> [_ _ _ _ _ _ _ _ _ _ w511 _ _ _ _ _ _ _ _ _ _ _ _ _ _ _ _ _ w642 _ _ w718 _ _]
            tunnel: w411 -> [_ _ _ _ _ _ _ w466 _ _ _ _ _ _ _ _ _ _ _ _ _ _ _ _ _ _ _ _ _ _ _ _ _ _]
            tunnel: w410 -> [_ _ _ _ _ _ _ _ _ _ _ _ _ _ _ _ _ _ _ _ _ _ _ _ _ _ _ w629 _ _ _ _ _ w747]
            tunnel: w409 -> [w422 _ _ _ _ _ _ w462 w494 _ _ _ w525 _ _ _ _ _ w565 _ _ _ w600 w610 _ _ _ _ w637 w687 w710 _ w740 _]
            tunnel: w408 -> [w419 _ _ _ _ _ _ w461 _ _ w513 _ w524 _ _ _ _ _ _ w570 w584 w589 _ _ _ w624 w628 _ _ _ w707 w729 w736 _]
            frame Default {
              n135 = call-poly "DatabaseHand_Get.vi"("name"=w420, "Database RefNum in"=w422) -> ("error out"=w423:errorcluster, "value"=w421:string)  [unwired: 3 in, 5 out]
              n136 = case shown="Error" w423 {
                tunnel: w427 -> [w429 _]
                tunnel: [w429 w434] -> w426
                tunnel: [w428 w430] -> w425
                tunnel: w424 -> [_ w433]
                tunnel: w420 -> [_ w432]
                tunnel: w421 -> [w428 _]
                tunnel: w419 -> [_ w431]
                frame No Error {
                }
                frame Error {
                  n137 = call "DHE_send_custom.vi"("valid params"=w433, "args"=w432, "fd"=w431) -> ("error IO"=w434:errorcluster, "str result"=w430:string)  [unwired: 1 in, 6 out]
                  n138 = Unbundle By Name(w434) -> ()  [unwired: 1 out]
                }
              }
            }
            frame "binning" {
              n139 = call "GEOM_GetModifiers.vi"("error in (no error)"=w441) -> ("error out"=w440:errorcluster, "GEOM_modifiers"=w439:T8)  [unwired: 9 out]
              n140 = Unbundle By Name(w439) -> ("Binning.x"=w438:u32, "Binning.y"=w437:u32)
              n141 = Format Into String(format string="x %d y %d", w438, w437) -> (resulting string=w435:string)  [unwired: 2 in, 1 out]
            }
            frame "bpp" {
              n142 = call "DHE_Getbpp.vi"() -> ("DHE_bpp"=w443:i32)  [unwired: 9 out]
              n143 = Format Into String(w443) -> (resulting string=w442:string)  [unwired: 3 in, 1 out]
            }
            frame "readmode", "readoutmode" {
              n144 = call "DHE_GetReadMode.vi"() -> ("DHE_ReadMode"=w445:string)  [unwired: 9 out]
            }
            frame "readmodes" {
              n145 = call "GEOM_GetAvailableReadModes.vi"() -> ("info"=w447:string)  [unwired: 1 in, 10 out]
            }
            frame "idle", "idlemode" {
              n146 = Unbundle By Name(w451) -> ("idlemode"=w450:bool)
              n147 = Append True/False String(1:w450, 2:"no" ("false string"), 3:"yes" ("true string")) -> (0:w452:string)  [unwired: 1 out]
            }
            frame "power" {
              n148 = Unbundle By Name(w457) -> ("power"=w460:bool)
              n149 = Append True/False String(1:w460, 2:"no" ("false string"), 3:"yes" ("true string")) -> (0:w456:string)  [unwired: 1 out]
            }
            frame "shutter" {
              n150 = Scan From String(format string="%s", input string=w466) -> (output 1=w464:string)  [unwired: 2 in, 4 out]
              n151 = To Lower Case(string=w464) -> (all lower case string=w463:string)
              n152 = case shown="Default" w463 {
                tunnel: w469 -> [_ w477]
                tunnel: [w470 w476] -> w468
                tunnel: w462 -> [w471 _]
                tunnel: w461 -> [_ w475]
                frame "type" {
                  n153 = call-poly "DatabaseHand_Get.vi"("name"="shutt_type", "Database RefNum in"=w471) -> ("value"=w470:string)  [unwired: 3 in, 6 out]
                }
                frame Default {
                  n154 = call "DHE_get_shutter_pos.vi"("fd"=w475) -> ("shutter"=w473:i32, "error out"=w474:errorcluster)  [unwired: 1 in, 12 out]
                  n155 = case shown="No Error" w474 {
                    tunnel: w477 -> [w487 w489]
                    tunnel: [w485 w488] -> w476
                    tunnel: w473 -> [w483 _]
                    frame No Error {
                      n156 = Greater Than 0?(x=w483) -> (x > 0?=w478:bool)
                      n157 = Equal To 0?(x=w483) -> (x = 0?=w482:bool)
                      n158 = Select(t="closed" ("false string"), s=w482, f="error" ("t")) -> (s? t:f=w481:string)
                      n159 = Append True/False String(1:w478, 2:w481, 3:"open" ("true string")) -> (0:w485:string)  [unwired: 1 out]
                      n160 = Bundle By Name(cluster=w487, "shutter"=w478) -> (w484:T5)
                      n161 = call "DHE_SetControllerStatus.vi"("ControllerStatus"=w484) -> ()  [unwired: 1 in, 10 out]
                    }
                    frame Error {
                      n162 = Unbundle By Name(w489) -> ("shutter"=w492:bool)
                      n163 = Append True/False String(1:w492, 2:"closed" ("false string"), 3:"open" ("true string")) -> (0:w488:string)  [unwired: 1 out]
                    }
                  }
                }
              }
            }
            frame "firmware" {
              n164 = call-poly "DatabaseHand_Get.vi"("name"="dhe_firmware", "Database RefNum in"=w494) -> ("value"=w493:string)  [unwired: 3 in, 6 out]
            }
            frame "gainspeed" {
              n165 = Unbundle By Name(w499) -> ("gain"=w502:u8, "speed"=w501:u8)
              n166 = Format Into String(format string="%d %d", w502, w501) -> (resulting string=w497:string)  [unwired: 2 in, 1 out]
            }
            frame "pixeltime", "pixtime" {
              n167 = Search 1D Array(1D array=w511, element="-unit") -> (index of element=w509:i32)  [unwired: 1 out]
              n168 = call "DHE_get_pixel_time.vi"("fd in"=w513) -> ("pix_time (usecs)"=w512:sgl)  [unwired: 1 in, 13 out]
              n169 = Greater Or Equal To 0?(x=w509) -> (x >= 0?=w508:bool)
              n170 = Format Into String(format string="%6.2f", w512) -> (resulting string=w504:string)  [unwired: 2 in, 1 out]
              n171 = Select(t="[ us/pix]", s=w508, f="") -> (s? t:f=w506:string)
              n172 = Concatenate Strings(w504, w506) -> (w503:string)
            }
            frame "gain" {
              n173 = Unbundle By Name(w518) -> ("gain"=w520:u8)
              n174 = Format Into String(format string="%d", w520) -> (resulting string=w516:string)  [unwired: 2 in, 1 out]
            }
            frame "expcode" {
              n175 = call "DHE_get_expcode.vi"("fd"=w524) -> ("expcode"=w522:i32, "error out"=w523:errorcluster)  [unwired: 1 in, 12 out]
              n176 = case shown="No Error" w523 {
                tunnel: [w531 w537] -> w526
                tunnel: w525 -> [w530 w536]
                tunnel: w522 -> [w529 _]
                tunnel: "expcode" ("name") -> [w528 w533]
                frame No Error {
                  n177 = call-poly "DatabaseHand_Set.vi"("name"=w528, "value"=w529, "Database RefNum in"=w530) -> ()  [unwired: 5 in, 4 out]
                  n178 = Format Into String(format string="%d", w529) -> (resulting string=w531:string)  [unwired: 2 in, 1 out]
                }
                frame Error {
                  n179 = call-poly "DatabaseHand_Get.vi"("default value"=1, "name"=w533, "Database RefNum in"=w536) -> ("value"=w534:i32)  [unwired: 2 in, 6 out]
                  n180 = Format Into String(format string="%d", w534) -> (resulting string=w537:string)  [unwired: 2 in, 1 out]
                }
              }
            }
            frame "speed" {
              n181 = Unbundle By Name(w541) -> ("speed"=w543:u8)
              n182 = Format Into String(format string="%d", w543) -> (resulting string=w539:string)  [unwired: 2 in, 1 out]
            }
            frame "artifdata", "artificialdata" {
              n183 = Unbundle By Name(w546) -> ("artifdata"=w549:bool)
              n184 = Append True/False String(1:w549, 2:"no" ("false string"), 3:"yes" ("true string")) -> (0:w544:string)  [unwired: 1 out]
            }
            frame "expasync" {
              n185 = call "DHE_GetAsyncExp.vi"() -> ("DHE_asyncexp"=w550:bool)  [unwired: 9 out]
              n186 = Append True/False String(1:w550, 2:"no" ("false string"), 3:"yes" ("true string")) -> (0:w551:string)  [unwired: 1 out]
            }
            frame "appendid" {
              n187 = call "DHE_GetAppendID.vi"() -> ("DHE_asyncexp"=w555:bool)  [unwired: 9 out]
              n188 = Append True/False String(1:w555, 2:"no" ("false string"), 3:"yes" ("true string")) -> (0:w556:string)  [unwired: 1 out]
            }
            frame "artifpatterns" {
              n189 = call "DHE_GetArtifPatterns.vi"() -> ("DHE_ArtifPatterns"=w560:string)  [unwired: 9 out]
            }
            frame "artifpattern" {
              n190 = call-poly "DatabaseHand_Get.vi"("default value"="none", "name"="artifpatt", "Database RefNum in"=w565) -> ("value"=w563:string)  [unwired: 2 in, 6 out]
            }
            frame "autoshutter" {
              n191 = call "DHE_get_autoshutter.vi"("fd in"=w570, "error in (no error)"=w569) -> ("autoshutter"=w567:bool, "error out"=w568:errorcluster)  [unwired: 12 out]
              n192 = case shown="No Error" w568 {
                tunnel: w572 -> [w578 w580]
                tunnel: [w576 w579] -> w571
                tunnel: w567 -> [w576 _]
                frame No Error {
                  n193 = Bundle By Name(cluster=w578, "autoshutter"=w576) -> (w577:T5)
                  n194 = call "DHE_SetControllerParams.vi"("ControllerStatus"=w577) -> ()  [unwired: 1 in, 10 out]
                }
                frame Error {
                  n195 = Unbundle By Name(w580) -> ("autoshutter"=w579:bool)
                }
              }
              n196 = Append True/False String(1:w571, 2:"no" ("false string"), 3:"yes" ("true string")) -> (0:w573:string)  [unwired: 1 out]
            }
            frame "samplings" {
              n197 = call "DHE_get_samplings.vi"("fd in"=w584, "error in (no error)"=w583) -> ("autoshutter"=w581:string, "error out"=w582:errorcluster)  [unwired: 12 out]
            }
            frame "autoclear" {
              n198 = call "DHE_get_autoclear.vi"("fd in"=w589, "error in (no error)"=w588) -> ("autoclear"=w586:bool, "error out"=w587:errorcluster)  [unwired: 12 out]
              n199 = case shown="No Error" w587 {
                tunnel: w590 -> [w596 w597]
                tunnel: [w594 w598] -> w585
                tunnel: w586 -> [w594 _]
                frame No Error {
                  n200 = Bundle By Name(cluster=w596, "autoclear"=w594) -> (w595:T5)
                  n201 = call "DHE_SetControllerParams.vi"("ControllerStatus"=w595) -> ()  [unwired: 1 in, 10 out]
                }
                frame Error {
                  n202 = Unbundle By Name(w597) -> ("autoclear"=w598:bool)
                }
              }
              n203 = Append True/False String(1:w585, 2:"no" ("false string"), 3:"yes" ("true string")) -> (0:w591:string)  [unwired: 1 out]
            }
            frame "autohandleclear", "handleclear" {
              n204 = call-poly "DatabaseHand_Get.vi"("default value"=TRUE, "name"="autohandleclear", "Database RefNum in"=w600) -> ("value"=w599:bool)  [unwired: 2 in, 6 out]
              n205 = Append True/False String(1:w599, 2:"no" ("false string"), 3:"yes" ("true string")) -> (0:w604:string)  [unwired: 1 out]
            }
            frame "arm", "armed" {
              n206 = call-poly "DatabaseHand_Get.vi"("default value"=FALSE, "name"="armed", "Database RefNum in"=w610) -> ("value"=w607:bool)  [unwired: 2 in, 6 out]
              n207 = Append True/False String(1:w607, 2:"no" ("false string"), 3:"yes" ("true string")) -> (0:w612:string)  [unwired: 1 out]
            }
            frame "config", "controllerconfig" {
              n208 = call "DHE_GetControllerConfig.vi"() -> ("ControllerConfigCluster"=w618:T3)  [unwired: 11 out]
              n209 = stacked-sequence {
                tunnel: [_ w620] -> w617
                tunnel: w618 -> [w619 _]
                frame #0 {
                  "ControllerConfigCluster" <- w619
                }
                frame #1 {
                  n210 = control-ref of="ControllerConfigCluster"() -> (w620:refnum<vi>)
                }
              }
              n211 = call "CMN_Struct2Str.vi"("Cluster Ref"=w617) -> ("Controls Text"=w615:string)  [unwired: 2 in, 7 out]
            }
            frame "controller_info", "controllerinfo", "hardware_info", "info" {
              n212 = call "DHE_get_controller_info.vi"("fd"=w624, "error in (no error)"=w622) -> ("info"=w623:string, "error out"=w621:errorcluster)  [unwired: 12 out]
            }
            frame "channel_info", "link_info", "pci_info" {
              n213 = call "DHE_get_link_info.vi"("fd"=w628, "error in (no error)"=w626) -> ("info"=w627:string, "error out"=w625:errorcluster)  [unwired: 12 out]
            }
            frame "state" {
            }
            frame "timing", "timinginfo" {
              w633 = "\n"
              n214 = stacked-sequence {
                tunnel: [_ w667] -> w638
                tunnel: w637 -> [w665 _]
                tunnel: [w663 _] -> w634
                tunnel: [w659 _] -> w632
                frame #0 {
                  n215 = call "DHE_GetTimingInfo.vi"("Database RefNum out"=w665) -> ("exposure_overhead"=w661:dbl, "seqs_overhead"=w662:dbl, "Timing"=→"Timing":T2)  [unwired: 8 out]
                  n216 = Format Into String(format string="exp_overhead= %6.3f", w661) -> (resulting string=w659:string)  [unwired: 2 in, 1 out]
                  n217 = Format Into String(format string="seq_overhead= %6.3f", w662) -> (resulting string=w663:string)  [unwired: 2 in, 1 out]
                }
                frame #1 {
                  n218 = control-ref of="Timing"() -> (w667:refnum<vi>)
                }
              }
              n219 = Search 1D Array(1D array=w642, element="-unit") -> (index of element=w640:i32)  [unwired: 1 out]
              n220 = call "CMN_Struct2Str.vi"("Cluster Ref"=w638) -> ("Controls Text"=w643:string)  [unwired: 2 in, 7 out]
              n221 = Greater Or Equal To 0?(x=w640) -> (x >= 0?=w639:bool)
              n222 = case shown="False" w639 {
                tunnel: w643 -> [w645 w651]
                tunnel: [w645 w648] -> w635
                tunnel: ["" " [s]"] -> w631
                tunnel: w632 -> [_ _]
                frame False {
                }
                frame True {
                  n223 = for {
                    tunnel: w651 -> [w658]
                    tunnel: string[] [" [us]", " [us]", " [us]", " [us]", " [pix]", " [s]"] -> [w655] mode=indexing
                    shift-right: [w654] -> w648
                    shift-left: "" -> [w653]
                    i -> [w657]
                    n224 = Pick Line(multi-line string=w658, line index=w657) -> (output string=w656:string)  [unwired: 1 out]
                    n225 = Concatenate Strings(w653, w656, w655, "\n") -> (w654:string)
                  }
                }
              }
              n226 = Concatenate Strings(w632, w631, w633, w634, w631, w633, w635) -> (w636:string)
            }
            frame "sampling" {
              n227 = call-poly "DatabaseHand_Get.vi"("default value"=FALSE, "name"="inversecds", "Database RefNum in"=w687) -> ("value"=w684:bool, "Database RefNum out"=w680:T1)  [unwired: 2 in, 5 out]
              n228 = call-poly "DatabaseHand_Get.vi"("name"="logic_proc", "Database RefNum in"=w680) -> ("value"=w678:string, "Database RefNum out"=w675:T1)  [unwired: 3 in, 5 out]
              n229 = Select(t="inverse", s=w684, f="normal") -> (s? t:f=w681:string)
              n230 = call-poly "DatabaseHand_Get.vi"("default value"=FALSE, "name"="cont_read", "Database RefNum in"=w675) -> ("value"=w674:bool, "Database RefNum out"=w668:T1)  [unwired: 2 in, 5 out]
              n231 = To Upper Case(1:w678) -> (0:w689:string)
              n232 = case shown="\"MULTFRAMES\"" w689 {
                selector: w689 -> [_ _ _ _ w705]
                tunnel: [w691 "single" "singframe" w697 w705] -> w669
                tunnel: w681 -> [w690 _ _ _ _]
                tunnel: w668 -> [_ _ _ w703 _]
                frame "COADD", "DCS", "FOWLER" {
                  n233 = Concatenate Strings("CDS ", w690) -> (w691:string)
                }
                frame "CCD", "OPTICAL", "SINGLE" {
                }
                frame "CCDIV" {
                }
                frame "MULTFRAMES" {
                  w700 = "pixsampling" ("name")
                  n234 = call-poly "DatabaseHand_Get.vi"("default value"=FALSE, "name"=w700, "Database RefNum in"=w703) -> ("value"=w701:bool)  [unwired: 2 in, 6 out]
                  n235 = call <vilib>:"Space Constant.vi"() -> ("String"=w696:string)
                  n236 = Select(t=w700, s=w701, f="") -> (s? t:f=w695:string)
                  n237 = Concatenate Strings("multframes", w696, w695) -> (w698:string)
                  n238 = call <vilib>:"Trim Whitespace.vi"("string"=w698) -> ("trimmed string"=w697:string)  [unwired: 1 in]
                }
                frame Default {
                }
              }
              n239 = Select(t=" continuous", s=w674, f="") -> (s? t:f=w671:string)
              n240 = Concatenate Strings(w669, w671) -> (w670:string)
            }
            frame "min_exptime", "minexptime" {
              n241 = flat-sequence {
                tunnel: w706 -> [w712]
                tunnel: w707 -> [w713]
                tunnel: w710 -> [w715]
                tunnel: [w714] -> w708
                frame #0 {
                  n242 = call "DHE_get_frame_time.vi"("fd in"=w713, "error in (no error)"=w712) -> ()  [unwired: 14 out]
                }
                frame #1 {
                  n243 = call "DHE_CalcExptime.vi"("DHE_DBSRef"=w715) -> ("min_exp_time"=w714:dbl)  [unwired: 1 in, 9 out]
                }
              }
              n244 = Format Into String(format string="%8.6f", w708) -> (resulting string=w709:string)  [unwired: 2 in, 1 out]
            }
            frame "frame_time", "hard_read_time" {
              n245 = Search 1D Array(1D array=w718, element="-unit") -> (index of element=w723:i32)  [unwired: 1 out]
              n246 = call "DHE_get_frame_time.vi"("fd in"=w729, "error in (no error)"=w728) -> ("frame_time"=w726:dbl, "error out"=w727:errorcluster)  [unwired: 12 out]
              n247 = Greater Or Equal To 0?(x=w723) -> (x >= 0?=w722:bool)
              n248 = Select(t=" [ s]", s=w722, f="") -> (s? t:f=w720:string)
              n249 = Number To Fractional String(number=w726, precision (6)=i16 3) -> (F-format string=w716:string)  [unwired: 2 out]
              n250 = Concatenate Strings(w716, w720) -> (w717:string)
            }
            frame "read_time" {
              n251 = call "DHE_get_frame_time.vi"("fd in"=w736, "error in (no error)"=w735) -> ("frame_time"=w730:dbl, "error out"=w734:errorcluster)  [unwired: 12 out]
              n252 = Unbundle By Name(w734) -> ("status"=w732:bool)
              n253 = Greater Than 0?(x=w730) -> (x > 0?=w733:bool)
              n254 = And(x=w733, y=w732) -> (x .and. y?=w731:bool)
              n255 = case shown="True" w731 {
                tunnel: w740 -> [w743 _]
                tunnel: [w742 w744] -> w737
                tunnel: w730 -> [_ w744]
                frame False {
                  n256 = call "DHE_GetTimingInfo.vi"("Database RefNum out"=w743) -> ("Timing"=w741:T2)  [unwired: 10 out]
                  n257 = Unbundle By Name(w741) -> ("DET_READ_TIME"=w742:sgl)
                }
                frame True {
                  n258 = call "DHE_GetTimingInfo.vi"() -> ("Timing"=w746:T2)  [unwired: 1 in, 10 out]
                  n259 = Bundle By Name(cluster=w746, "DET_READ_TIME"=w744) -> (w745:T2)
                  n260 = call "DHE_SetTimingInfo.vi"("Timing"=w745) -> ()  [unwired: 1 in, 10 out]
                }
              }
              n261 = Number To Fractional String(number=w737, precision (6)=i16 3) -> (F-format string=w738:string)  [unwired: 2 out]
            }
            frame "" {
            }
          }
        }
        frame "status" {
          n262 = call "DHE_GetStatus.vi"() -> ("DHE_Status"=w749:string)  [unwired: 9 out]
          n263 = Scan From String(format string="%s", input string=w749) -> (output 1=w755:string)  [unwired: 2 in, 4 out]
          n264 = call "DHE_GetModuleName.vi"() -> ("DHE_ModuleName"=w750:string)  [unwired: 9 out]
          n265 = Equal?(x=w755, y="NOT") -> (x = y?=w753:bool)
          n266 = call "CMN_testmessage.vi"("message  in"=w749) -> ("ERROR"=w751:bool)  [unwired: 1 in, 9 out]
          n267 = Or(x=w751, y=w753) -> (x .or. y?=w752:bool)
          n268 = case shown="False" w752 {
            tunnel: w749 -> [w764 w795]
            tunnel: [w763 w795] -> w757
            tunnel: w750 -> [w761 _]
            frame False {
              w762 = " " ("string")
              n269 = call "DHE_GetImgState.vi"() -> ("DHE_ImgState"=w760:T11)  [unwired: 9 out]
              n270 = case shown="\"Initializing\"" w760 {
                tunnel: "state =" -> [w768 w772 w775 w778 w781 w784 w787 w790 w793 _]
                tunnel: [w767 w770 w773 w776 w779 w782 w785 w788 w791 "initializing"] -> w765
                frame "Idle", Default {
                  n271 = Concatenate Strings(w768, "idle" ("string")) -> (w767:string)
                }
                frame "Exposing" {
                  n272 = Concatenate Strings(w772, "exposing" ("string")) -> (w770:string)
                }
                frame "Paused" {
                  n273 = Concatenate Strings(w775, "paused" ("string")) -> (w773:string)
                }
                frame "AbortExp" {
                  n274 = Concatenate Strings(w778, "AbortExp" ("string")) -> (w776:string)
                }
                frame "Reading" {
                  n275 = Concatenate Strings(w781, "reading" ("string")) -> (w779:string)
                }
                frame "AbortRead" {
                  n276 = Concatenate Strings(w784, "abortread" ("string")) -> (w782:string)
                }
                frame "FinishedReading" {
                  n277 = Concatenate Strings(w787, "finishedreading" ("string")) -> (w785:string)
                }
                frame "Resetting" {
                  n278 = Concatenate Strings(w790, "reseting" ("string")) -> (w788:string)
                }
                frame "Reducing" {
                  n279 = Concatenate Strings(w793, "reducing" ("string")) -> (w791:string)
                }
                frame "Initializing" {
                }
              }
              n280 = Concatenate Strings(w761, w762, w764, w762, w765) -> (w763:string)
            }
            frame True {
            }
          }
        }
        frame "efficiency" {
          n281 = call "CMN_Efficiency.vi"("Action"=enum16{"ADD", "CLEAR", "GET"}."GET") -> ("efficency"=w799:dbl)  [unwired: 3 in, 7 out]
          n282 = Number To Fractional String(number=w799) -> (F-format string=w798:string)  [unwired: 3 out]
        }
        frame "modinfo", "version" {
          n283 = Current VI's Path() -> (path=w804:path)
          n284 = call "CMN_modinfo.vi"("error in (no error)"=w802, "full"=TRUE, "caller path"=w804) -> ("INFO"=w801:string)  [unwired: 8 out]
        }
        frame "initmacro" {
          n285 = call "DHE_GetInitMacro.vi"() -> ("DHE_InitMacro"=w806:path)  [unwired: 9 out]
          n286 = Path To String(path=w806) -> (string=w807:string)
        }
        frame "macro_dir", "macrodir" {
          n287 = call "DHE_GetMacroDir.vi"() -> ("DHE_MacroDir"=w810:path)  [unwired: 9 out]
          n288 = Path To String(path=w810) -> (string=w811:string)
        }
        frame "fpainfo" {
          n289 = Search 1D Array(1D array=w820, element="-full") -> (index of element=w818:i32)  [unwired: 1 out]
          n290 = Greater Or Equal To 0?(x=w818) -> (x >= 0?=w817:bool)
          n291 = case shown="True" w817 {
            tunnel: ["" w830] -> w816
            frame False {
            }
            frame True {
              n292 = call "DHE_GetFPAname.vi"() -> ("DHE_FPAname"=w826:string)  [unwired: 9 out]
              n293 = String To Path(string=w826) -> (path=w832:path)
              n294 = Strip Path(path=w832) -> (name=w828:string)  [unwired: 1 out]
              n295 = File/Directory Info(path=w832) -> (error out=w833:errorcluster)  [unwired: 1 in, 6 out]
              n296 = Concatenate Strings("database_path/FPA/" ("string"), w828) -> (w827:string)
              n297 = Select(t=w827, s=w833, f=w826) -> (s? t:f=w825:string)
              n298 = Concatenate Strings("file: " ("string"), w825, "\n") -> (w830:string)
            }
          }
          n299 = call "GEOM_GetFPAINFO.vi"("error in (no error)"=w823) -> ("error out"=w822:errorcluster, "info"=w815:string)  [unwired: 9 out]
          n300 = Concatenate Strings(w816, w815) -> (w814:string)
        }
        frame "detinfo" {
          n301 = Scan From String(format string="%d", input string=w837) -> (output 1=w835:i32)  [unwired: 2 in, 4 out]
          n302 = call "GEOM_GetDETNFO.vi"("error in (no error)"=w841, "detnum"=w835) -> ("error out"=w838:errorcluster, "info"=w839:string)  [unwired: 8 out]
        }
        frame "detector_format", "detformat" {
          n303 = call "GEOM_CallGeometry.vi"("Command"="GET DETFORMAT", "error in (no error)"=w845) -> ("ImmedReplyString"=w842:string, "error out"=w844:errorcluster)  [unwired: 12 out]
        }
        frame "ampinfo" {
          n304 = call "DHE_GetReadMode.vi"() -> ("DHE_ReadMode"=w850:string)  [unwired: 9 out]
          n305 = call <vilib>:"Space Constant.vi"() -> ("String"=w849:string)
          n306 = Concatenate Strings(w850, w849, w848) -> (w847:string)
          n307 = call "GEOM_GetStrAmps.vi"("args"=w847) -> ("amps"=w852:string)  [unwired: 2 in, 8 out]
        }
        frame "dettype" {
          n308 = call "DHE_GetControllerConfig.vi"() -> ("ControllerConfigCluster"=w858:T3)  [unwired: 11 out]
          n309 = Unbundle By Name(w858) -> ("Detector Type"=w857:string)
          n310 = To Upper Case(1:w857) -> (0:w856:string)
        }
        frame "normalize", "normalize_coadds" {
          n311 = call-poly "DatabaseHand_Get.vi"("default value"=FALSE ("Normalize"), "name"="normalize_coadds" ("value"), "Database RefNum in"=w867) -> ("value"=w862:bool)  [unwired: 2 in, 6 out]
          n312 = Append True/False String(1:w862, 2:"no" ("false string"), 3:"yes" ("true string")) -> (0:w859:string)  [unwired: 1 out]
        }
        frame "memrule" {
          n313 = call-poly "DatabaseHand_Get.vi"("default value"="releasediff" ("value"), "name"="memrule" ("value"), "Database RefNum in"=w873) -> ("value"=w868:string)  [unwired: 2 in, 6 out]
        }
        frame "interlock", "interlocks" {
          n314 = Scan From String(format string="%s", input string=w884) -> (remaining string=w885:string, output 1=w883:string)  [unwired: 2 in, 3 out]
          n315 = Search 1D Array(1D array=w880, element="-all") -> (index of element=w878:i32)  [unwired: 1 out]
          n316 = Greater Or Equal To 0?(x=w878) -> (x >= 0?=w877:bool)
          n317 = call <vilib>:"Trim Whitespace.vi"("string"=w885) -> ("trimmed string"=w882:string)  [unwired: 1 in]
          n318 = case shown="\"state\"" w883 {
            selector: w883 -> [w889 _ _]
            tunnel: w882 -> [_ w901 w910]
            tunnel: w877 -> [w891 _ _]
            tunnel: [w890 w904 w909] -> w876
            tunnel: w875 -> [w888 w903 w907]
            tunnel: [w887 w902 w906] -> w874
            frame Default {
              n319 = case shown="False" w891 {
                tunnel: [w894 w899] -> w890
                tunnel: w889 -> [w895 _]
                tunnel: w888 -> [w893 w898]
                tunnel: [w892 w897] -> w887
                frame False {
                  n320 = call "DHE_InterlockMngr.vi"("error in (no error)"=w893, "Enum"=T4."find", "command"=w895) -> ("error out"=w892:errorcluster, "response"=w894:string)  [unwired: 1 in, 6 out]
                }
                frame True {
                  n321 = call "DHE_InterlockMngr.vi"("error in (no error)"=w898, "Enum"=T4."getall") -> ("error out"=w897:errorcluster, "response"=w899:string)  [unwired: 2 in, 6 out]
                }
              }
            }
            frame "state" {
              n322 = call "DHE_InterlockMngr.vi"("error in (no error)"=w903, "Enum"=T4."getall", "command"=w901) -> ("error out"=w902:errorcluster, "response"=w904:string)  [unwired: 1 in, 6 out]
            }
            frame "", "all", "getall" {
              n323 = call "DHE_InterlockMngr.vi"("error in (no error)"=w907, "Enum"=T4."getall" ("f"), "command"=w910) -> ("error out"=w906:errorcluster, "response"=w909:string)  [unwired: 1 in, 6 out]
            }
          }
        }
        frame Default {
          w914 = "_UNDEF_" ("default value")
          # "first, try getting it from the database,\nif not found, ask it to the current hardware,\nin case it is a specific hardware parameter.\nIf the hardware does not know it,\nreturn an error"
          n324 = call-poly "DatabaseHand_Get.vi"("default value"=w914, "name"=w911, "Database RefNum in"=w919) -> ("error out"=w917:errorcluster, "value"=w915:string)  [unwired: 2 in, 5 out]
          n325 = Unbundle By Name(w917) -> ("status"=w916:bool)
          n326 = Equal?(x=w914, y=w915) -> (x = y?=w913:bool)
          n327 = Or(x=w913, y=w916) -> (x .or. y?=w912:bool)
          n328 = case shown="True" w912 {
            tunnel: w924 -> [w926 w936]
            tunnel: [w926 w935] -> w923
            tunnel: [w927 w934] -> w922
            tunnel: w921 -> [w925 w932]
            tunnel: [w925 w931] -> w920
            tunnel: w911 -> [_ w929]
            tunnel: w918 -> [_ w928]
            tunnel: w915 -> [w927 _]
            frame False {
            }
            frame True {
              n329 = case shown="Default" w929 {
                selector: w929 -> [w937 _]
                tunnel: w928 -> [_ _]
                tunnel: [w937 w939] -> w930
                frame "", "?", "help" {
                }
                frame Default {
                  n330 = Scan From String(format string="%s", input string="Command + switches") -> (remaining string=w938:string, output 1=w942:string)  [unwired: 2 in, 3 out]
                  n331 = Concatenate Strings("get_" ("string"), w942, w938) -> (w939:string)
                }
              }
              n332 = call "DHE_send_custom.vi"("valid params"=string[] ["image.<..> [?]", "dhe.<..> [?]", "obs.<..> [?]", "status", "fpainfo", "detinfo <detnum>", "initmacro", "macrodir", "dettype", "modinfo", "efficiency"], "error in (no error)"=w936, "args"=w930, "fd"=w932) -> ("error IO"=w935:errorcluster, "fd out"=w931:i32)  [unwired: 6 out]
              n333 = Unbundle By Name(w935) -> ("source"=w934:string)
            }
          }
        }
      }
    }
    frame Error {
      n334 = Unbundle By Name(w945) -> ("source"=w944:string)  [unwired: 1 out]
    }
  }
  "refnum out" <- w10
  "error out" <- w8
  "response" <- w4
